vi "Adder.vi"() -> ()   [LabVIEW 2013]
panel:
  out "C":dbl
  in  "Sum":bool
  in  "B":dbl
  in  "A":dbl
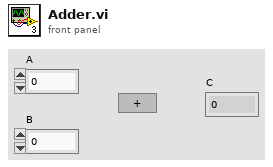
[diagram p1: front panel]
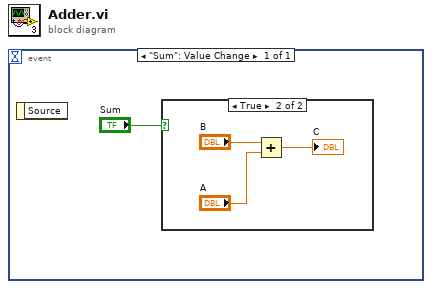
[diagram p0: block diagram]
diagram:
  n1 = event shown="[0] \"Sum\": Value Change" {
    selector: _ -> [_]
    dyn-events: _ -> [_]
    timeout: _ -> [_]
    event "Sum": Value Change {
      n2 = event-data() -> ()  [unwired: 1 in, 1 out]
      n3 = case shown="True" "Sum" {
        frame False {
        }
        frame True {
          n4 = Add(x="B", y="A") -> (x+y=→"C":dbl)
        }
      }
    }
  }
